vi "Handle Exit.vi"(8 "error in (no error)":errorcluster, 9 "Stop Argument":T1, 10 "Admin in":refnum<class "Delacor_lib_QMH_Module Admin.lvclass">) -> (0 "error out":errorcluster, 3 "Wait for Module to stop?":bool)   [LabVIEW 2024, in "Power Supply.lvlib"]
doc: "This VI handles the Exit Message for a DQMH Singleton module. \n\nThis VI determines if the message was received via the Stop Request or not. If the Exit message was received via the Request Event to Stop the module then there is no need to send the Stop Request again. If it was not, then the Stop Request needs to be fired so the Event Handling Loop can stop.\n\nThis VI also hides the Main.vi Front Panel, this is to ensure that the module stays in memory until the very last step in the Main.vi which is to close the front panel.\n_____\nBased on Delacor QMH Project Template 3.1.0.34."
uses:
  Power Supply.lvlib
  <vilib>/Delacor/Delacor QMH/Libraries/Module Admin_class/Delacor_lib_QMH_Module Admin.lvclass
  Stop Argument--cluster.ctl
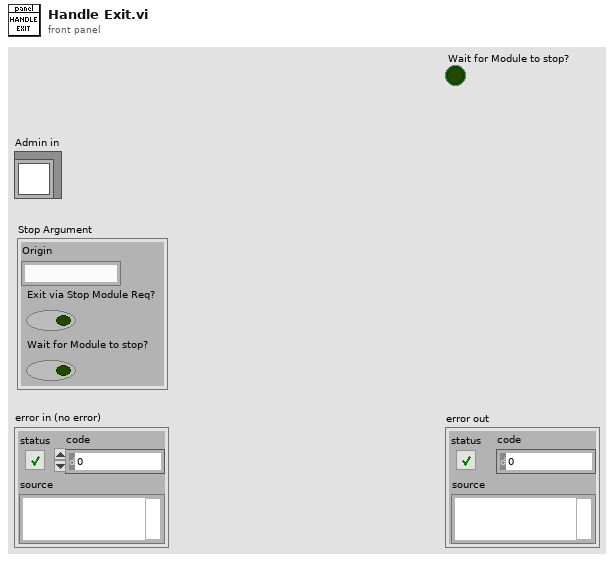
[diagram p1: front panel]
types:
  T1 = typedef "Power Supply.lvlib/Stop Argument--cluster.ctl" = cluster{"Origin":string, "Exit via Stop Module Req?":bool, "Wait for Module to stop?":bool}
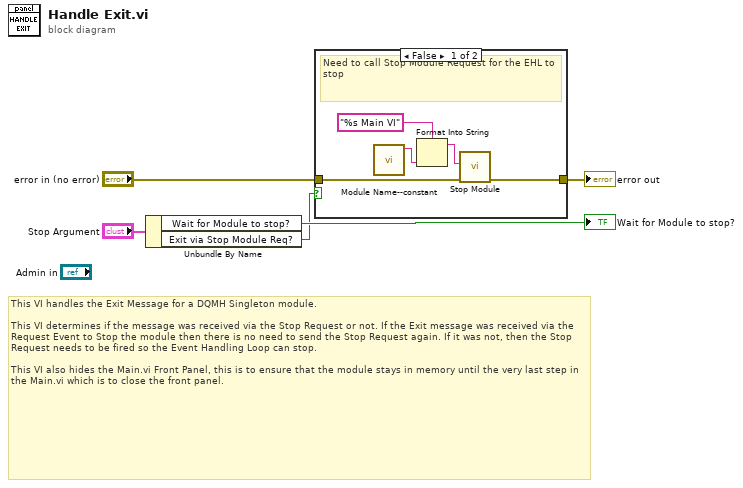
[diagram p0: block diagram]
diagram:
  # "This VI handles the Exit Message for a DQMH Singleton module. \n\nThis VI determines if the message was received via the Stop Request or not. If the Exit message was received via the Request Event to Stop the module then there is no need to send the Stop Request again. If it was not, then the Stop Request needs to be fired so the Event Handling Loop can stop.\n\nThis VI also hides the Main.vi Front Panel, this is to ensure that the module stays in memory until the very last step in the Main.vi which is to close the front panel."
  n1 = Unbundle By Name("Stop Argument") -> ("Wait for Module to stop?"=→"Wait for Module to stop?":bool, "Exit via Stop Module Req?"=w2:bool)
  n2 = case "Exit came from Stop Module Request?" shown="False" w2 {
    tunnel: [w8 w11] -> w4
    tunnel: "error in (no error)" -> [w6 w11]
    frame False {
      # "Need to call Stop Module Request for the EHL to stop"
      n3 = call "Module Name--constant.vi"() -> ("Module Name"=w7:string)  [unwired: 11 in]
      n4 = Format Into String(format string="%s Main VI", w7) -> (resulting string=w9:string)  [unwired: 2 in, 1 out]
      n5 = call "Stop Module.vi"("error in (no error)"=w6, "Origin"=w9) -> ("error out"=w8:errorcluster)  [unwired: 9 in]
    }
    frame True {
      # "no need to call Stop Module Request again."
    }
  }
  "error out" <- w4
